vi "DWT_morlet.vi"(6 "dt":dbl=0.01, 7 "1D Real input":dbl[](array[numeric])=[-0.12679116993991574, 1.0193746308657807, -0.09052850382765222, 0.8042744316138584, 1.4808495240538322, 1.4291018069524823, 1.907980569429116, 1.4444030818238436, 1.4250374884460215, 1.58618677339917, 1.2418812976353384, 0.06934243553306585, 0.7029921341129483, 0.2782545942983345, 0.1394399612276337, 0.34779060464719935, 0.4439893646282308, 0.27733249967907214, -0.19706440881629483, -0.3628828613463365, 0.40742276472198286, -0.17006282090809255, 0.6133579235877548, 0.135225005473686, 1.2239060367091286, 1.3030478750158971, 1.7552098340714117, 0.9237689415025249, 1.1806608708634987, 0.8449898593246244, 1.9174780618729304, 1.7840917064159778, 1.1728058423770225, 1.62153061196214, -0.272656310860608, -0.5558007349304581, -0.2959380241573938, -1.4300133213604551, -0.6823822866643512, -0.91572439933541, -0.5669602443605319, -0.7587378967054472, -0.8549457794853906, -0.5286303747846421, -0.5251425475661455, -0.7383335058141725, -0.8894339293623567, -0.5095844142979015, -0.03366004962887231, -0.6726284692596878, 0.814510855805496, 0.43359760803524083, 0.6608576403261218, 0.4161416450987375, 0.5517723125739475, 0.5798229474199644, -0.4912224295292563, -0.23530828902401035, -1.0480526583129628, -1.7707539107927446, -0.45994426286484524, -1.261500851578112, -1.9870080202457276, -1.8875038544595575, -2.366116694057184, -0.5783874187761651, -0.8920666066594337, -0.09405261653471741, -0.7751223671526339, -1.0944419076129368, -0.14005875931722112, 0.48987264941225483, -0.3676808301547359, 1.1587151094942756, 1.2670010184574225, 1.217787716962798, 0.565459483140733, 0.9087280535389326, 0.5939835710531244, 1.1017983215191332, 1.6650248633852214, 0.3553867707228626, 0.2753505228614388, 0.00903992491248723, 0.49792164659785537, -0.616346978147716, -0.630721259664082, 0.014299524970964872, 0.480700475302101, -0.6951626078729354, -1.0661467333723311, 0.3011749805002055, 0.6408264916230577, -0.29558883407774084, 1.0748658387415926, 1.6251075589788795, 1.6543652350157318, 1.3596309066154832, 0.7307529223553038, 1.2749760701978792, 1.0904296229985855, 2.155020822538927, 1.2623484530797549, 1.1496055457853402, 0.844557726791297, 0.6395670246468422, 0.02451901217593988, -0.7977563246290675, -0.3088887306171158, -0.36149790118779973, -0.18506023518919767, -0.6590292722336561, -0.43177219770058933, -0.8762086585429315, -0.7205677382596106, -0.09636822077327098, -0.5327650799543888, -0.3289978059655324, 0.48172164002821183, -0.05325070621040778, 1.0565530051794245, 0.3683362411324411, 0.9499221878080258, 0.2981621528978346, 1.1468623385778964, -0.34617334693401014, -0.1386666097898116, -0.5666387111824267, -0.3348657678600956, -0.8240355555671138, -0.9321141609392499, -1.5294700968704524, -2.572121647649663, -1.3050926473915148, -1.6616233056293233, -1.241752101388613, -1.4187627680937274, -1.3509798526619665, -0.4215366529572309, -1.2967019469830074, -0.35293187277868177, -0.5904743644700152, -0.2917239985095182, -0.47483335692682804, 0.46180597035652504, 0.9840630091285274, 1.299382197706025, 0.43619754791853427, 0.32695105622941406, 0.5911085332330913, 0.1628226777454026, -0.34635582105481316, -0.2681363765456337, -0.7818888801571826, -0.18136698271320434, -0.4298364717378451, -0.9487826007092731, -1.1737256088430341, 0.14283138519098712, -0.39453950887377787, 0.3546479425290055, 0.23298902952377146, -0.30380160693537406, 0.808348817755246, 0.736202238584211, 1.512267622218586, 1.2365429410301585, 1.727413622876901, 2.543874302822961, 1.2079375646221377, 2.2292137440248276, 1.2440179132437799, 1.6682015726886066, 0.13464608391118882, 0.2913489646300522, 0.15990820077122458, 0.662428421060336, -0.29037544700528195, 0.06614244071467446, -0.3382332191980665, -0.23666225114045192, -0.4295749317256162, -0.09265859638971652, 0.17975061431408368, 0.8536137863756864, 0.9453632762875829, 0.10501908244828517, 1.9388160694121452, 0.5373318864662969, 0.530494871186602, 1.2001058047784747, 1.0286115657640555, 1.0072460834189787, 1.2282318440312243, 0.8830821412839315, 0.9190465913844457, -0.6115135906212075, 0.6178965974331141, -0.5568347377689267, -0.3482444967847503, -0.9079988262952523, -1.6969820147031682, -1.6501111349985482, -1.6348540433665955, 0.22573099951580766, -1.4972471308996655, -1.2911833594242639, -0.45307152385800303, -1.5851251387443859, -1.1249610156485135, -0.727130599354048, 0.3351713628428937, 0.211800860828244, -0.8552385428474392, 0.623008044838545, 0.5227772532313715, -0.21955991775566186, -0.7042140586981246, 0.8555341729414853, -0.2712824196457748, -0.573880829671195, -0.3535477891310561, -1.5147969910466226, -1.4679572589437409, -0.8610096035147358, -0.7873014895781181, -0.3835366613360319, -0.6402446092361875, -1.360917499164956, -1.2530674615165958, -0.32269694023733575, -1.000270314298563, 0.2767342644167296, 0.5011463548424178, 0.8905439234425838, 1.427471229960774, 1.686886460756448, 0.8169252416945002, 0.7930026992817341, 0.6895596339385863, 0.4789952846078418, 0.30345373064448267, 0.299838197907486, 1.2467363214472353, 0.6559131742913148, -0.08786188046771715, -0.9246223905422474, -0.3784066679268775, -0.5897014580421297, -0.37375301367134106, -0.5963723252989973, 0.013998650298599147, 0.05800660194203755, 0.2597093941840749, 1.5369611125101166, 1.1329936565910785]) -> (1 "Wavelet plot":dbl[][](graph))   [LabVIEW 2011]
uses:
  <vilib>/Analysis/2dsp.llb/Real FFT.vi
  <vilib>/Analysis/2dsp.llb/Inverse Complex FFT.vi
  <vilib>/Analysis/NI_AALPro.lvlib
panel:
  out "Input":dbl[](graph)=[-0.12679116993991574, 1.0193746308657807, -0.09052850382765222, 0.8042744316138584, 1.4808495240538322, 1.4291018069524823, 1.907980569429116, 1.4444030818238436, 1.4250374884460215, 1.58618677339917, 1.2418812976353384, 0.06934243553306585, 0.7029921341129483, 0.2782545942983345, 0.1394399612276337, 0.34779060464719935, 0.4439893646282308, 0.27733249967907214, -0.19706440881629483, -0.3628828613463365, 0.40742276472198286, -0.17006282090809255, 0.6133579235877548, 0.135225005473686, 1.2239060367091286, 1.3030478750158971, 1.7552098340714117, 0.9237689415025249, 1.1806608708634987, 0.8449898593246244, 1.9174780618729304, 1.7840917064159778, 1.1728058423770225, 1.62153061196214, -0.272656310860608, -0.5558007349304581, -0.2959380241573938, -1.4300133213604551, -0.6823822866643512, -0.91572439933541, -0.5669602443605319, -0.7587378967054472, -0.8549457794853906, -0.5286303747846421, -0.5251425475661455, -0.7383335058141725, -0.8894339293623567, -0.5095844142979015, -0.03366004962887231, -0.6726284692596878, 0.814510855805496, 0.43359760803524083, 0.6608576403261218, 0.4161416450987375, 0.5517723125739475, 0.5798229474199644, -0.4912224295292563, -0.23530828902401035, -1.0480526583129628, -1.7707539107927446, -0.45994426286484524, -1.261500851578112, -1.9870080202457276, -1.8875038544595575, -2.366116694057184, -0.5783874187761651, -0.8920666066594337, -0.09405261653471741, -0.7751223671526339, -1.0944419076129368, -0.14005875931722112, 0.48987264941225483, -0.3676808301547359, 1.1587151094942756, 1.2670010184574225, 1.217787716962798, 0.565459483140733, 0.9087280535389326, 0.5939835710531244, 1.1017983215191332, 1.6650248633852214, 0.3553867707228626, 0.2753505228614388, 0.00903992491248723, 0.49792164659785537, -0.616346978147716, -0.630721259664082, 0.014299524970964872, 0.480700475302101, -0.6951626078729354, -1.0661467333723311, 0.3011749805002055, 0.6408264916230577, -0.29558883407774084, 1.0748658387415926, 1.6251075589788795, 1.6543652350157318, 1.3596309066154832, 0.7307529223553038, 1.2749760701978792, 1.0904296229985855, 2.155020822538927, 1.2623484530797549, 1.1496055457853402, 0.844557726791297, 0.6395670246468422, 0.02451901217593988, -0.7977563246290675, -0.3088887306171158, -0.36149790118779973, -0.18506023518919767, -0.6590292722336561, -0.43177219770058933, -0.8762086585429315, -0.7205677382596106, -0.09636822077327098, -0.5327650799543888, -0.3289978059655324, 0.48172164002821183, -0.05325070621040778, 1.0565530051794245, 0.3683362411324411, 0.9499221878080258, 0.2981621528978346, 1.1468623385778964, -0.34617334693401014, -0.1386666097898116, -0.5666387111824267, -0.3348657678600956, -0.8240355555671138, -0.9321141609392499, -1.5294700968704524, -2.572121647649663, -1.3050926473915148, -1.6616233056293233, -1.241752101388613, -1.4187627680937274, -1.3509798526619665, -0.4215366529572309, -1.2967019469830074, -0.35293187277868177, -0.5904743644700152, -0.2917239985095182, -0.47483335692682804, 0.46180597035652504, 0.9840630091285274, 1.299382197706025, 0.43619754791853427, 0.32695105622941406, 0.5911085332330913, 0.1628226777454026, -0.34635582105481316, -0.2681363765456337, -0.7818888801571826, -0.18136698271320434, -0.4298364717378451, -0.9487826007092731, -1.1737256088430341, 0.14283138519098712, -0.39453950887377787, 0.3546479425290055, 0.23298902952377146, -0.30380160693537406, 0.808348817755246, 0.736202238584211, 1.512267622218586, 1.2365429410301585, 1.727413622876901, 2.543874302822961, 1.2079375646221377, 2.2292137440248276, 1.2440179132437799, 1.6682015726886066, 0.13464608391118882, 0.2913489646300522, 0.15990820077122458, 0.662428421060336, -0.29037544700528195, 0.06614244071467446, -0.3382332191980665, -0.23666225114045192, -0.4295749317256162, -0.09265859638971652, 0.17975061431408368, 0.8536137863756864, 0.9453632762875829, 0.10501908244828517, 1.9388160694121452, 0.5373318864662969, 0.530494871186602, 1.2001058047784747, 1.0286115657640555, 1.0072460834189787, 1.2282318440312243, 0.8830821412839315, 0.9190465913844457, -0.6115135906212075, 0.6178965974331141, -0.5568347377689267, -0.3482444967847503, -0.9079988262952523, -1.6969820147031682, -1.6501111349985482, -1.6348540433665955, 0.22573099951580766, -1.4972471308996655, -1.2911833594242639, -0.45307152385800303, -1.5851251387443859, -1.1249610156485135, -0.727130599354048, 0.3351713628428937, 0.211800860828244, -0.8552385428474392, 0.623008044838545, 0.5227772532313715, -0.21955991775566186, -0.7042140586981246, 0.8555341729414853, -0.2712824196457748, -0.573880829671195, -0.3535477891310561, -1.5147969910466226, -1.4679572589437409, -0.8610096035147358, -0.7873014895781181, -0.3835366613360319, -0.6402446092361875, -1.360917499164956, -1.2530674615165958, -0.32269694023733575, -1.000270314298563, 0.2767342644167296, 0.5011463548424178, 0.8905439234425838, 1.427471229960774, 1.686886460756448, 0.8169252416945002, 0.7930026992817341, 0.6895596339385863, 0.4789952846078418, 0.30345373064448267, 0.299838197907486, 1.2467363214472353, 0.6559131742913148, -0.08786188046771715, -0.9246223905422474, -0.3784066679268775, -0.5897014580421297, -0.37375301367134106, -0.5963723252989973, 0.013998650298599147, 0.05800660194203755, 0.2597093941840749, 1.5369611125101166, 1.1329936565910785]
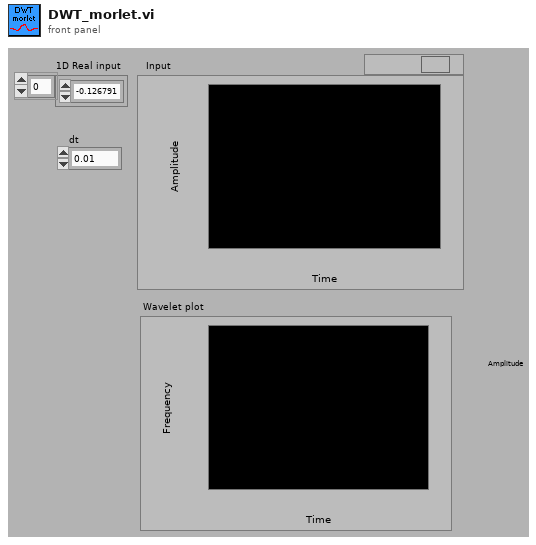
[diagram p1: front panel]
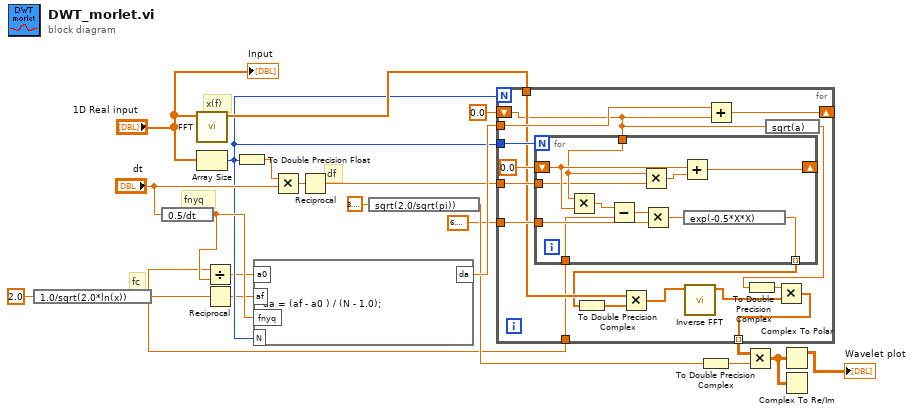
[diagram p0: block diagram]
diagram:
  # "fc"
  # "fnyq"
  # "x(f)"
  # "df"
  n1 = expression code="1.0/sqrt(2.0*ln(x))"(2.0) -> (w3:dbl)
  n2 = expression code="0.5/dt"("dt") -> (w10:dbl)
  n3 = call-poly <vilib>:"FFT.vi"("X"="1D Real input") -> ("FFT {X}"=w11:cdb[])  [unwired: 2 in, 8 out]
  n4 = Array Size(array="1D Real input") -> (size(s)=w8:i32)
  n5 = Divide(x=w3, y=w10) -> (x/y=w7:dbl)
  n6 = Reciprocal(x=w3) -> (1/x=w1:dbl)
  n7 = To Double Precision Float(number=w8) -> (double precision float=w21:dbl)
  n8 = formula code="da = (af - a0 ) / (N - 1.0);"("a0"=w7, "fnyq"=w10, "N"=w8, "af"=w1) -> ("da"=w18:dbl)
  n9 = Multiply(x=w21, y="dt") -> (x*y=w20:dbl)
  n10 = Reciprocal(x=w20) -> (1/x=w17:dbl)
  n11 = expression code="sqrt(2.0/sqrt(pi))"(3.141592653589793) -> (w14:dbl)
  n12 = for {
    N: w8 -> [_]
    shift-right: [w37] -> _
    shift-left: 0.0 -> [w29]
    tunnel: w18 -> [w36]
    tunnel: w8 -> [w35]
    tunnel: 6.283185307179586 -> [w33]
    tunnel: w17 -> [w32]
    tunnel: w11 -> [w31]
    tunnel: [w26] -> w15 mode=indexing
    tunnel: w3 -> [w22]
    n13 = for {
      N: w35 -> [_]
      shift-right: [w48] -> _
      shift-left: 0.0 -> [w46]
      tunnel: w29 -> [w45]
      tunnel: w33 -> [w47]
      tunnel: w32 -> [w39]
      tunnel: [w40] -> w23 mode=indexing
      tunnel: w22 -> [w42]
      n14 = Multiply(x=w45, y=w46) -> (x*y=w43:dbl)
      n15 = Subtract(x=w43, y=w42) -> (x-y=w41:dbl)
      n16 = Multiply(x=w45, y=w39) -> (x*y=w38:dbl)
      n17 = Multiply(x=w41, y=w47) -> (x*y=w44:dbl)
      n18 = Add(x=w46, y=w38) -> (x+y=w48:dbl)
      n19 = expression code="exp(-0.5*X*X)"(w44) -> (w40:dbl)
    }
    n20 = To Double Precision Complex(1:w23) -> (0:w30:cdb[])
    n21 = Multiply(x=w31, y=w30) -> (x*y=w25:cdb[])
    n22 = call-poly <vilib>:"Inverse FFT.vi"("FFT {X}"=w25) -> ("X"=w24:cdb[])  [unwired: 1 in, 9 out]
    n23 = Add(x=w36, y=w29) -> (x+y=w37:dbl)
    n24 = expression code="sqrt(a)"(w29) -> (w28:dbl)
    n25 = To Double Precision Complex(1:w28) -> (0:w27:cdb)
    n26 = Multiply(x=w27, y=w24) -> (x*y=w26:cdb[])
  }
  n27 = To Double Precision Complex(1:w14) -> (0:w13:cdb)
  n28 = Multiply(x=w15, y=w13) -> (x*y=w12:cdb[][])
  n29 = Complex To Polar(r * e^(i*theta)=w12) -> (r=→"Wavelet plot":dbl[][])  [unwired: 1 out]
  n30 = Complex To Re/Im(x + iy=w12) -> ()  [unwired: 2 out]
  "Input" <- "1D Real input"
